vi "Stop Core.vi"(10 "final error code":i32, 11 "Table View in":refnum<class "Table View.lvclass">) -> (3 "Table View out":refnum<class "Table View.lvclass">)   [LabVIEW 2020, in "[V]Table View.lvlib" / "Table View.lvclass"]
doc: "(<B>Filename</B>: Actor Framework.lvlib:Actor.lvclass:Stop Core.vi)\n\nDefines what the actor does before it stops. Use the <B>final error code</B> input to determine whether the actor shut down in response to an error.\n\nBy default, this method passes the Stop message along to all auto-stop nested actors. A descendant class may override this method to define additional behavior, such as shutting down any processes the actor initiated in its override of the Actor Core method."
uses:
  Table View.lvclass
  Table View.lvclass/Table View.ctl
  Depden On/MVVM Framework/MVVM Abstruct View/MVVM Abstruct View/MVVM Abstruct View.lvclass
  <vilib>/HUASUI/MulListBox/MListBox.lvclass
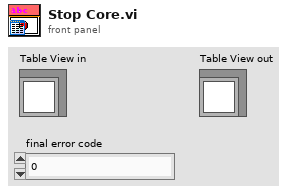
[diagram p1: front panel]
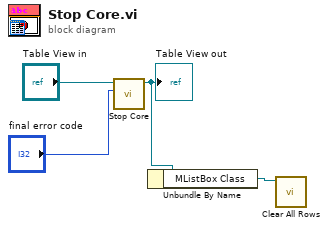
[diagram p0: block diagram]
diagram:
  n1 = call-parent "Stop Core.vi"("final error code"="final error code", "Abstruct View in"="Table View in") -> ("Abstruct View out"=w2:refnum<class "Table View.lvclass">)  [unwired: 9 in]
  "Table View out" <- w2
  n2 = Unbundle By Name(w2) -> ("MListBox Class"=w1:refnum<class "MListBox.lvclass">)
  n3 = call <vilib>:"Clear All Rows.vi"("Multicolumn ListBox in"=w1) -> ()  [unwired: 9 in, 2 out]
